vi "Julian Date Calculator.vi"() -> (2 "current time":timestamp, 3 "JD":ext=2446895.5 format="%_12f", 4 "tau (measured in Julian millenia)":dbl=-0.012729637234770705 format="%#_10g", 8 "LST [hh:mm:ss]":string="15:28:59.491", 10 "T (measured in Julian centuries)":ext=-0.12729637234770704996 format="%_12g", 13 "LST [Deg]":ext, 14 "LST [Hours]":ext, 15 "GST[0-360]":dbl=197.6931950962171 format="%#_9g")   [LabVIEW 2015]
panel:
  out "LST - GST in Hours":ext
  in  "Observer's Longitude":ext=105.2369444444 format="%#_10g"
  out "HMS Time":string="13:10:46.3668"
  out "GST [HA]":dbl=13.179546339747807
  out "GST":ext=-1678122.3068049038 format="%#_14f"
  # "Epoch J2000.0 correseponds to the Julian Date for Year 2000, Month 1 (Jan) and Day 1.5\n\nJDE = Julian Ephemeris Day corresponding to a given instant.\n\n                 JDE - 2451545.0\ntau      =     -------------------\n                      365250"
  # "These are MEAN Greenwich Sideral Time, not Apparent Greenwich Sidereal time which still\nrequires a correction for delta-psi nutation"
  # "NOAA Solar Position Calculator \nDefault Position for Boulder, CO is\n105 Degrees, 14 Min, 13 Sec West of Greenwich"
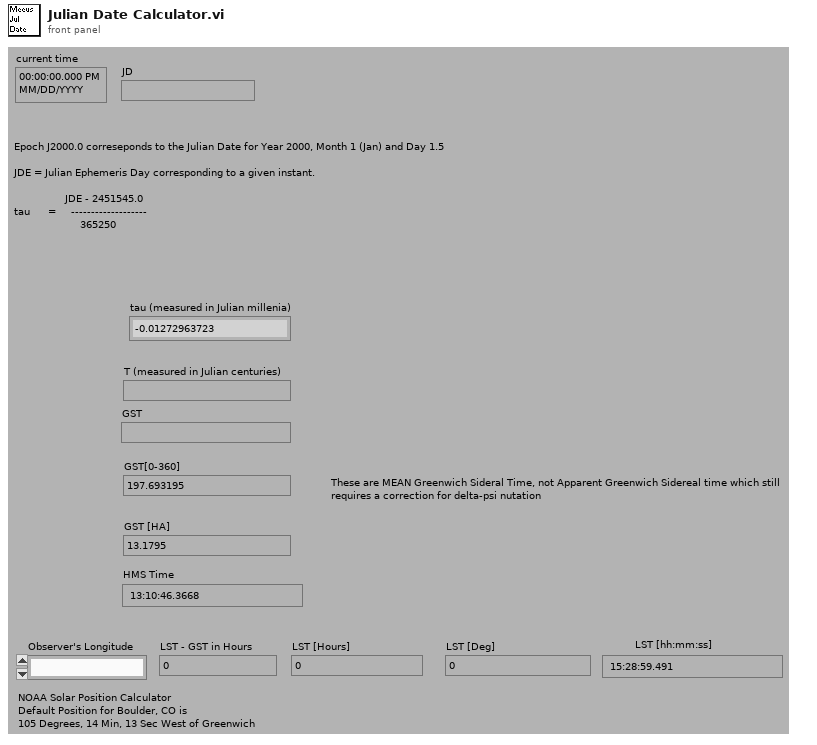
[diagram p1: front panel]
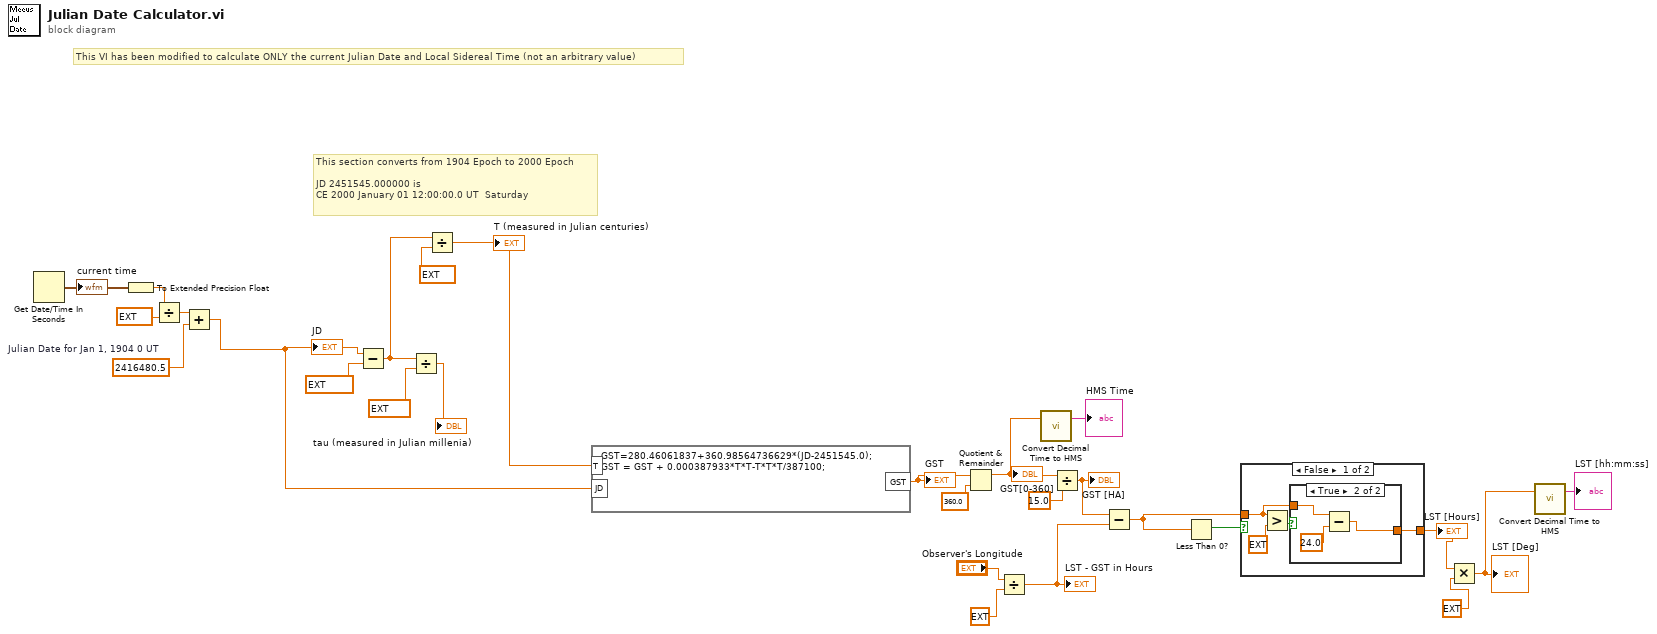
[diagram p0: block diagram]
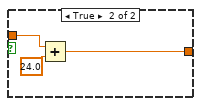
[diagram p3: hidden frame]
diagram:
  w2 = 2416480.5  # Julian Date for Jan 1, 1904 0 UT
  # "This VI has been modified to calculate ONLY the current Julian Date and Local Sidereal Time (not an arbitrary value)"
  # "This section converts from 1904 Epoch to 2000 Epoch\n\nJD 2451545.000000 is\nCE 2000 January 01 12:00:00.0 UT  Saturday"
  n1 = Get Date/Time In Seconds() -> (seconds since 1Jan1904=w6:timestamp)
  "current time" <- w6
  n2 = To Extended Precision Float(1:w6) -> (0:w5:ext)
  n3 = Divide(x=w5, y=ext 86400.0) -> (x/y=w3:ext)
  n4 = Add(x=w3, y=w2) -> (x+y=w1:ext)
  "JD" <- w1
  n5 = Subtract(x=w1, y=ext 2451545.0) -> (x-y=w23:ext)
  n6 = Divide(x=w23, y=ext 365250.0) -> (x/y=→"tau (measured in Julian millenia)":ext)
  n7 = Divide(x=w23, y=ext 36525.0) -> (x/y=w22:ext)
  "T (measured in Julian centuries)" <- w22
  n8 = formula code="GST=280.46061837+360.98564736629*(JD-2451545.0);\nGST = GST + 0.000387933*T*T-T*T*T/387100;"("T"=w22, "JD"=w1) -> ("GST"=w20:dbl)
  "GST" <- w20
  n9 = Quotient & Remainder(x=w20, y=360.0) -> (x-y*floor(x/y)=w17:dbl)  [unwired: 1 out]
  "GST[0-360]" <- w17
  n10 = Divide(x="Observer's Longitude", y=ext 15.0) -> (x/y=w13:ext)
  "LST - GST in Hours" <- w13
  n11 = call "Convert Decimal Time to HMS.vi"("Decimal Time"=w17) -> ("HMS Time"=→"HMS Time":string)  [unwired: 2 out]
  n12 = Divide(x=w17, y=15.0) -> (x/y=w14:dbl)
  "GST [HA]" <- w14
  n13 = Subtract(x=w14, y=w13) -> (x-y=w11:ext)
  n14 = Less Than 0?(x=w11) -> (x < 0?=w12:bool)
  n15 = case shown="False" w12 {
    tunnel: w11 -> [w29 w37]
    tunnel: [w28 w36] -> w10
    frame False {
      n16 = Greater?(x=w29, y=ext 24.0) -> (0:w30:bool)
      n17 = case shown="True" w30 {
        tunnel: w29 -> [w32 w34]
        tunnel: [w32 w33] -> w28
        frame False {
        }
        frame True {
          n18 = Subtract(x=w34, y=24.0) -> (x-y=w33:ext)
        }
      }
    }
    frame True {
      n19 = Add(x=w37, y=24.0) -> (x+y=w36:ext)
    }
  }
  "LST [Hours]" <- w10
  n20 = Multiply(x=w10, y=ext 15.0) -> (x*y=w8:ext)
  "LST [Deg]" <- w8
  n21 = call "Convert Decimal Time to HMS.vi"("Decimal Time"=w8) -> ("HMS Time"=→"LST [hh:mm:ss]":string)  [unwired: 2 out]
